vi "Control_Gate.vi"(8 "error in (no error)":errorcluster, 9 "Control/Anti-control ?":bool, 10 "CtrlLine in":refnum<class "CtrlLine.lvclass">, 11 "QuWire in":refnum<class "QuWire.lvclass">) -> (0 "error out":errorcluster, 2 "CtrlLine out":refnum<class "CtrlLine.lvclass">, 3 "QuWire out":refnum<class "QuWire.lvclass">)   [LabVIEW 2020, in "QuWire.lvclass"]
uses:
  QuWire.lvclass
  CtrlLine/CtrlLine.lvclass
  QuWire.lvclass/QuWire.ctl
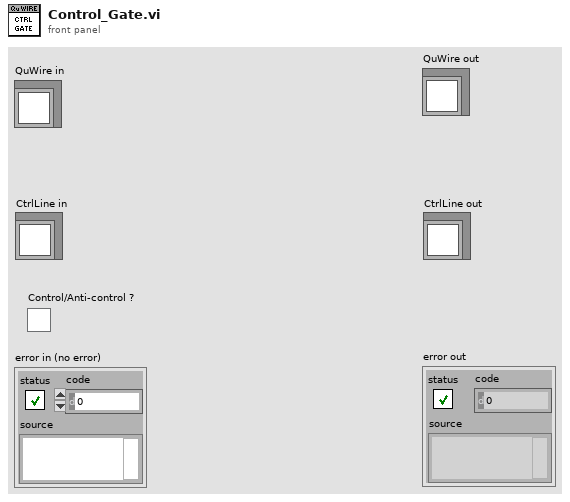
[diagram p1: front panel]
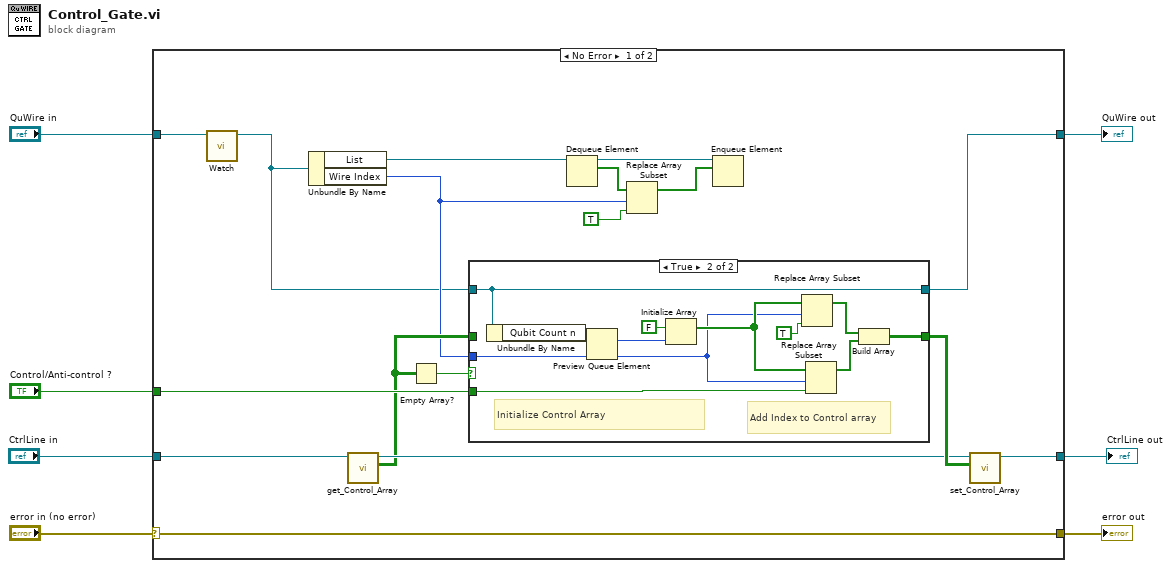
[diagram p0: block diagram]
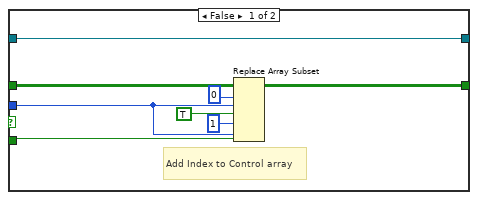
[diagram p2: hidden frame]
diagram:
  n1 = case shown="No Error" "error in (no error)" {
    selector: "error in (no error)" -> [w24 w46]
    tunnel: [w24 w46] -> w6
    tunnel: [w19 w45] -> w4
    tunnel: "QuWire in" -> [w20 w45]
    tunnel: "Control/Anti-control ?" -> [w22 _]
    tunnel: "CtrlLine in" -> [w23 w44]
    tunnel: [w21 w44] -> w1
    frame No Error {
      n2 = call "Watch.vi"("QuWire in"=w20) -> ("QuWire out"=w8:refnum<class "QuWire.lvclass">)  [unwired: 9 in, 1 out]
      n3 = Unbundle By Name(w8) -> ("List"=w17:refnum<queue>, "Wire Index"=w9:i32)
      n4 = call "get_Control_Array.vi"("CtrlLine in"=w23) -> ("Control Array"=w10:bool[][], "CtrlLine out"=w12:refnum<class "CtrlLine.lvclass">)  [unwired: 8 in, 1 out]
      n5 = Empty Array?(array=w10) -> (empty?=w11:bool)
      n6 = case shown="True" w11 {
        tunnel: w9 -> [w30 w38]
        tunnel: w22 -> [w29 w37]
        tunnel: [w26 w34] -> w18
        tunnel: w10 -> [w27 _]
        tunnel: w8 -> [w25 w33]
        tunnel: [w25 w33] -> w19
        frame False {
          # "Add Index to Control array"
          n7 = Replace Array Subset(array=w27, new element #1=TRUE ("new element/subarray"), index (row) #1=0 ("index (row)"), index (col) #1=w30, new element #2=w29, index (row) #2=1 ("index (row)"), index (col) #2=w30) -> (w26:bool[][])
        }
        frame True {
          # "Add Index to Control array"
          # "Initialize Control Array"
          n8 = Unbundle By Name(w33) -> ("Qubit Count n"=w43:refnum<queue>)
          n9 = Preview Queue Element(queue=w43) -> (element=w41:i32)  [unwired: 2 in, 3 out]
          n10 = Initialize Array(FALSE, w41) -> (w39:bool[])
          n11 = Replace Array Subset(array=w39, new element=TRUE ("new element/subarray"), index=w38) -> (w36:bool[])
          n12 = Replace Array Subset(array=w39, new element=w37, index=w38) -> (w35:bool[])
          n13 = Build Array(w36, w35) -> (w34:bool[][])
        }
      }
      n14 = Dequeue Element(queue=w17) -> (queue out=w16:refnum<queue>, element=w15:bool[])  [unwired: 2 in, 2 out]
      n15 = Replace Array Subset(array=w15, new element=TRUE ("new element/subarray"), index=w9) -> (w13:bool[])
      n16 = Enqueue Element(queue=w16, element=w13) -> ()  [unwired: 2 in, 3 out]
      n17 = call "set_Control_Array.vi"("Control Array"=w18, "CtrlLine in"=w12) -> ("CtrlLine out"=w21:refnum<class "CtrlLine.lvclass">)  [unwired: 8 in, 1 out]
    }
    frame Error {
    }
  }
  "error out" <- w6
  "QuWire out" <- w4
  "CtrlLine out" <- w1
